vi "Timestamp ISO8601.vi"() -> (3 "ISO 8601 Timestamp":string)   [LabVIEW 2020]
uses:
  <vilib>/regexp/Match Regular Expression.xnode
panel:
  in  "Time Stamp":timestamp
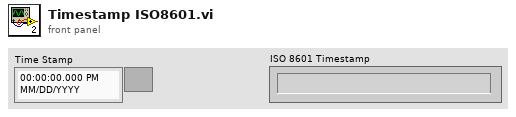
[diagram p1: front panel]
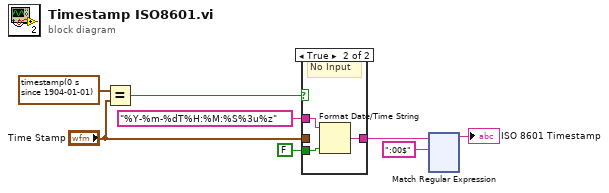
[diagram p0: block diagram]
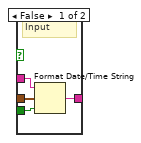
[diagram p2: hidden frame]
diagram:
  n1 = Equal?(x=timestamp(0 s since 1904-01-01) ("time stamp"), y="Time Stamp") -> (x = y?=w1:bool)
  n2 = case shown="True" w1 {
    tunnel: [w12 w15] -> w6
    tunnel: FALSE ("UTC format") -> [w11 w14]
    tunnel: "%Y-%m-%dT%H:%M:%S%3u%z" ("time format string (%c)") -> [w10 w13]
    tunnel: "Time Stamp" -> [w9 _]
    frame False {
      # "Input"
      n3 = Format Date/Time String(time format string (%c)=w10, seconds (now)=w9, UTC format=w11) -> (date/time string=w12:string)
    }
    frame True {
      # "No Input"
      n4 = Format Date/Time String(time format string (%c)=w13, UTC format=w14) -> (date/time string=w15:string)  [unwired: 1 in]
    }
  }
  n5 = xnode "Match Regular Expression"("input string"=w6, "regular expression"=":00$") -> ("before match"=→"ISO 8601 Timestamp":string)  [unwired: 4 in, 4 out]
